vi "扩展会话.vi"(8 "error in":errorcluster caption="error out", 10 "R_ID":u32=1844 format="0x%0x", 11 "T_ID":u32=1828 format="0x%x") -> (0 "error out":errorcluster caption="error in", 3 "OK":bool=TRUE)   [LabVIEW 2020]
panel:
  out "key":u16
  out "Out_Time":bool
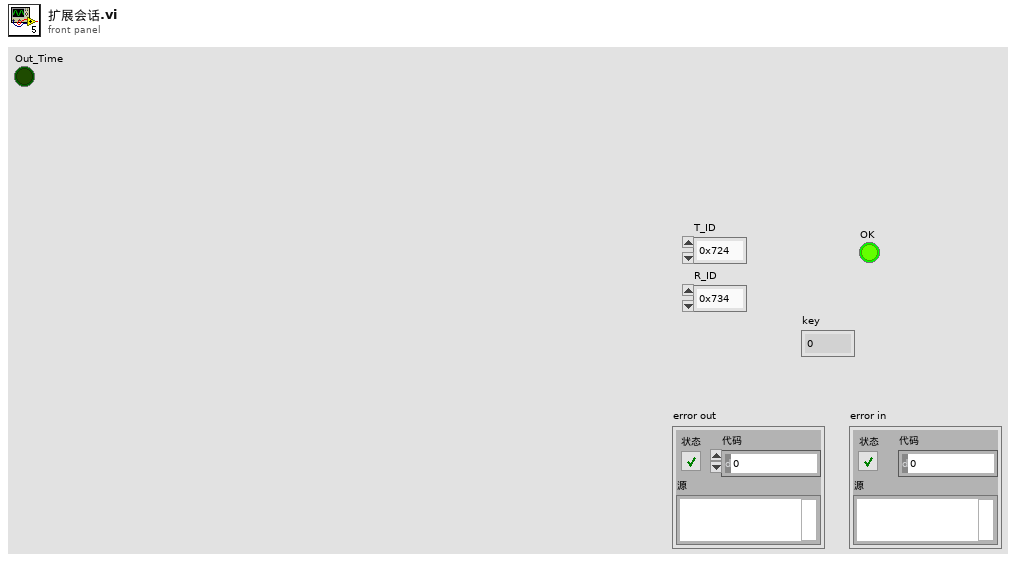
[diagram p1: front panel]
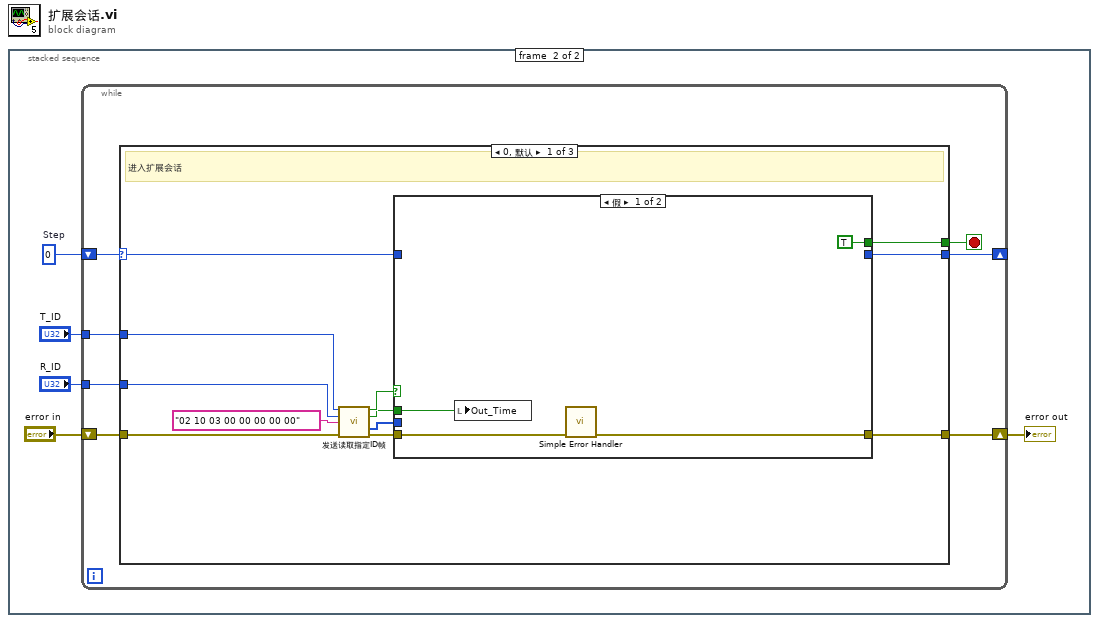
[diagram p0: block diagram]
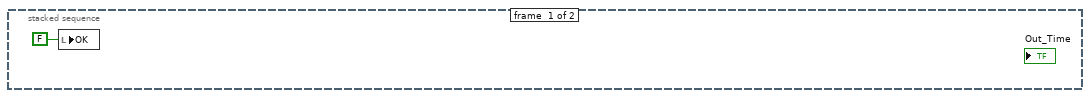
[diagram p2: hidden frame]
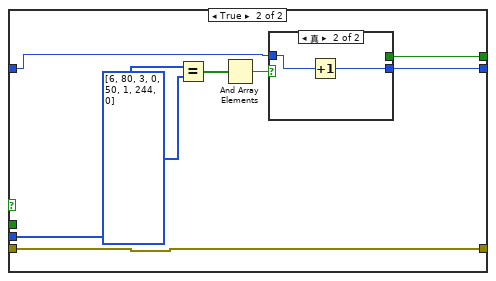
[diagram p3: hidden frame]
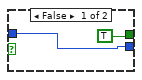
[diagram p4: hidden frame]
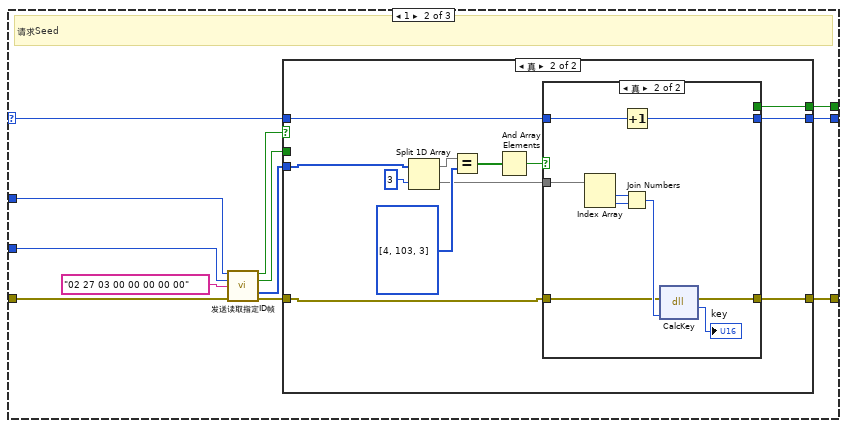
[diagram p5: hidden frame]
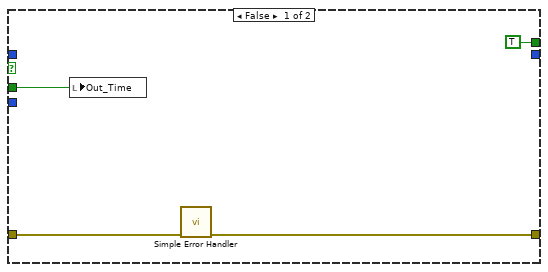
[diagram p6: hidden frame]
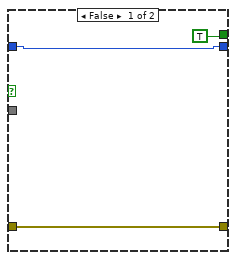
[diagram p7: hidden frame]
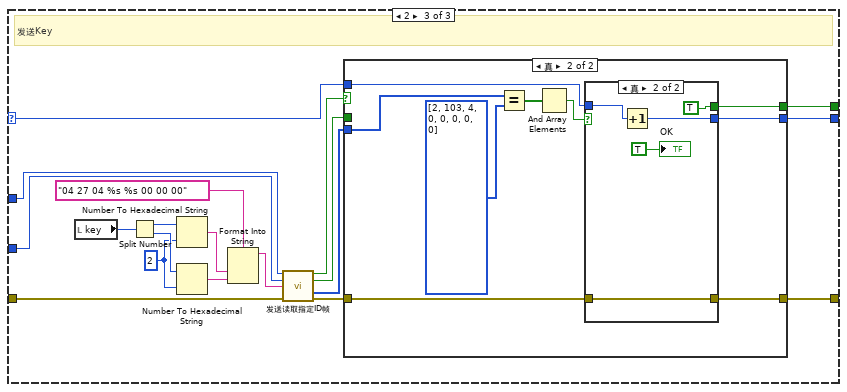
[diagram p8: hidden frame]
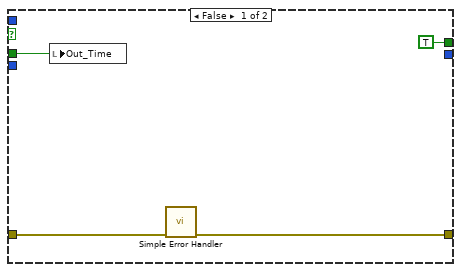
[diagram p9: hidden frame]
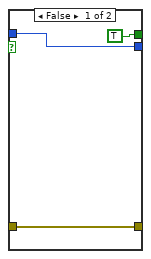
[diagram p10: hidden frame]
diagram:
  n1 = stacked-sequence {
    frame #0 {
      n2 = local write "OK"(FALSE ("OK")) -> ()
    }
    frame #1 {
      w4 = 0  # Step
      n3 = while {
        tunnel: "T_ID" -> [w13]
        tunnel: "R_ID" -> [w11]
        shift-right: [w7] -> _
        shift-left: w4 -> [w10]
        shift-right: [w8] -> w2
        shift-left: "error in" -> [w12]
        stop <- w9 stop-if-true
        n4 = case shown="0, 默认" w10 {
          selector: w10 -> [w15 w43 w91]
          tunnel: w13 -> [w25 w53 w100]
          tunnel: w12 -> [w24 w52 w99]
          tunnel: w11 -> [w23 w51 w98]
          tunnel: [w19 w47 w95] -> w9
          tunnel: [w17 w45 w93] -> w8
          tunnel: [w14 w42 w90] -> w7
          frame 0, Default {
            # "进入扩展会话"
            n5 = call "发送读取指定ID帧.vi"("T_ID"=w25, "R_ID"=w23, "CAN_Frame"="02 10 03 00 00 00 00 00", "error in (no error)"=w24) -> ("OK"=w21:bool, "Out_Time"=w20:bool, "Recive"=w16:u8[], "error out"=w18:errorcluster)  [unwired: 7 in, 1 out]
            n6 = case shown="假" w21 {
              tunnel: w20 -> [w29 _]
              tunnel: [TRUE w30] -> w19
              tunnel: w18 -> [w27 w37]
              tunnel: [w26 w37] -> w17
              tunnel: w16 -> [_ w36]
              tunnel: w15 -> [_ w34]
              tunnel: [_ w33] -> w14
              frame False {
                n7 = local write "Out_Time"(w29) -> ()
                n8 = call <vilib>:"Simple Error Handler.vi"("error in (no error)"=w27) -> ("error out"=w26:errorcluster)  [unwired: 4 in, 4 out]
              }
              frame True {
                n9 = Equal?(x=w36, y=u8[] [6, 80, 3, 0, 50, 1, 244, 0]) -> (x = y?=w32:bool[])
                n10 = And Array Elements(Boolean array=w32) -> (logical AND=w31:bool)
                n11 = case shown="真" w31 {
                  tunnel: w34 -> [w39 w41]
                  tunnel: [w39 w40] -> w33
                  tunnel: [TRUE _] -> w30
                  frame False {
                  }
                  frame True {
                    n12 = Increment(x=w41) -> (x+1=w40:i32)
                  }
                }
              }
            }
          }
          frame 1 {
            # "请求Seed"
            n13 = call "发送读取指定ID帧.vi"("T_ID"=w53, "R_ID"=w51, "CAN_Frame"="02 27 03 00 00 00 00 00", "error in (no error)"=w52) -> ("OK"=w49:bool, "Out_Time"=w48:bool, "Recive"=w44:u8[], "error out"=w46:errorcluster)  [unwired: 7 in, 1 out]
            n14 = case shown="真" w49 {
              tunnel: w48 -> [w57 _]
              tunnel: [TRUE w58] -> w47
              tunnel: w46 -> [w55 w62]
              tunnel: [w54 w61] -> w45
              tunnel: w44 -> [_ w67]
              tunnel: w43 -> [_ w60]
              tunnel: [_ w59] -> w42
              frame False {
                n15 = local write "Out_Time"(w57) -> ()
                n16 = call <vilib>:"Simple Error Handler.vi"("error in (no error)"=w55) -> ("error out"=w54:errorcluster)  [unwired: 4 in, 4 out]
              }
              frame True {
                n17 = Split 1D Array(array=w67, index=3 ("索引")) -> (first subarray=w65:u8[], second subarray=w64:u8[])
                n18 = Equal?(x=w65, y=u8[] [4, 103, 3]) -> (x = y?=w68:bool[])
                n19 = And Array Elements(Boolean array=w68) -> (logical AND=w63:bool)
                n20 = case shown="真" w63 {
                  tunnel: w64 -> [_ w81]
                  tunnel: w62 -> [w72 w77]
                  tunnel: [w72 w76] -> w61
                  tunnel: w60 -> [w71 w74]
                  tunnel: [w71 w73] -> w59
                  tunnel: [TRUE _] -> w58
                  frame False {
                  }
                  frame True {
                    n21 = Index Array(array=w81) -> (element #1=w80:u8, element #2=w79:u8)  [unwired: 2 in]
                    n22 = Increment(x=w74) -> (x+1=w73:i32)
                    n23 = Join Numbers(hi=w80, lo=w79) -> ((hi.lo)=w78:u16)
                    n24 = dll-call lib="PTH2^abs CUsersFeng项目HengLongtrunk性能试验台Sourcesdll安全算法.dll" fn="CalcKey"(error in=w77, "Seed"=w78) -> (error out=w76:errorcluster, "返回类型"=→"key":u16)  [unwired: 3 in, 1 out]
                  }
                }
              }
            }
          }
          frame 2 {
            w85 = i16 2 ("宽度(-)")
            # "发送Key"
            n25 = local read "key"() -> (w88:u16)
            n26 = Split Number(x=w88) -> (hi(x)=w87:u8, lo(x)=w86:u8)
            n27 = Number To Hexadecimal String(1:w85, 2:w87) -> (0:w84:string)
            n28 = Number To Hexadecimal String(1:w85, 2:w86) -> (0:w83:string)
            n29 = Format Into String(format string="04 27 04 %s %s 00 00 00" ("CAN_Frame"), w84, w83) -> (resulting string=w82:string)  [unwired: 2 in, 1 out]
            n30 = call "发送读取指定ID帧.vi"("T_ID"=w100, "R_ID"=w98, "CAN_Frame"=w82, "error in (no error)"=w99) -> ("OK"=w97:bool, "Out_Time"=w96:bool, "Recive"=w92:u8[], "error out"=w94:errorcluster)  [unwired: 7 in, 1 out]
            n31 = case shown="真" w97 {
              tunnel: w96 -> [w104 _]
              tunnel: [TRUE w105] -> w95
              tunnel: w94 -> [w102 w109]
              tunnel: [w101 w108] -> w93
              tunnel: w92 -> [_ w111]
              tunnel: w91 -> [_ w107]
              tunnel: [_ w106] -> w90
              frame False {
                n32 = local write "Out_Time"(w104) -> ()
                n33 = call <vilib>:"Simple Error Handler.vi"("error in (no error)"=w102) -> ("error out"=w101:errorcluster)  [unwired: 4 in, 4 out]
              }
              frame True {
                n34 = Equal?(x=w111, y=u8[] [2, 103, 4, 0, 0, 0, 0, 0]) -> (x = y?=w112:bool[])
                n35 = And Array Elements(Boolean array=w112) -> (logical AND=w110:bool)
                n36 = case shown="真" w110 {
                  tunnel: w109 -> [w116 w121]
                  tunnel: [w116 w121] -> w108
                  tunnel: w107 -> [w115 w120]
                  tunnel: [w115 w119] -> w106
                  tunnel: [TRUE TRUE] -> w105
                  frame False {
                  }
                  frame True {
                    n37 = Increment(x=w120) -> (x+1=w119:i32)
                    "OK" <- TRUE
                  }
                }
              }
            }
          }
        }
      }
      "error out" <- w2
    }
  }
